vi "GetExecutionMode.vi"(8 "error in (no error)":errorcluster, 11 "absolute custom device xml file":path) -> (0 "error out":errorcluster, 2 "execution mode":T1, 3 "absolute custom device xml file":path)   [LabVIEW 2016, in "VeriStandTestUtilities.lvlib"]
uses:
  VeriStandTestUtilities.lvlib
  <vilib>/NI Veristand/Custom Device API/Custom Device Execution Mode.ctl
  <vilib>/xml/Load XML File.vi
  <vilib>/xml/Close Reference(Node).vi
  <vilib>/xml/NI_XML.lvlib
  <vilib>/NI VeriStand/Custom Device API/Custom Device API.lvlib
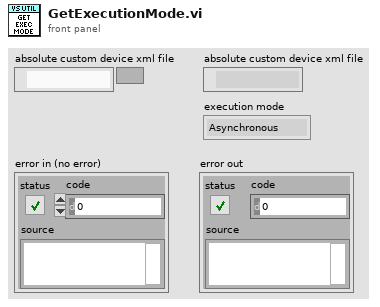
[diagram p1: front panel]
types:
  T1 = typedef "Custom Device API.lvlib/Custom Device Execution Mode.ctl" = enum16{"Asynchronous", "Inline HW Interface", "Inline Model Interface", "Inline Timing and Sync", "Asynchronous Timing and Sync"}
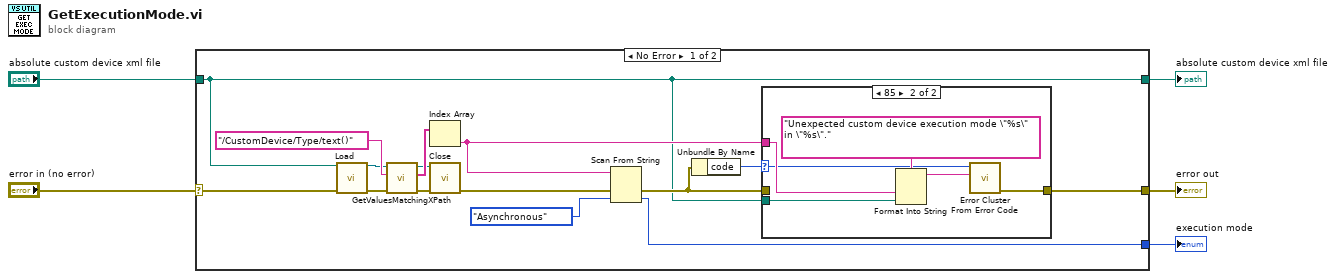
[diagram p0: block diagram]
diagram:
  n1 = case shown="No Error" "error in (no error)" {
    selector: "error in (no error)" -> [w20 w29]
    tunnel: "absolute custom device xml file" -> [w6 w28]
    tunnel: [w10 w29] -> w3
    tunnel: [w11 _] -> w2
    tunnel: [w6 w28] -> w1
    frame No Error {
      n2 = call-poly <vilib>:"Load.vi"("path to XML document"=w6, "error in (no error)"=w20) -> ("DOM document out"=w15:refnum<k20>, "error out"=w17:errorcluster)  [unwired: 11 in, 1 out]
      n3 = call "GetValuesMatchingXPath.vi"("error in (no error)"=w17, "XPath"="/CustomDevice/Type/text()", "XML refnum in"=w15) -> ("error out"=w18:errorcluster, "Values"=w16:string[], "XML refnum out"=w14:refnum<k20>)  [unwired: 6 in]
      n4 = Index Array(array=w16) -> (element=w7:string)  [unwired: 1 in]
      n5 = call-poly <vilib>:"Close.vi"("error in (no error)"=w18, "node"=w14) -> ("error out"=w12:errorcluster)  [unwired: 7 in]
      n6 = Scan From String(input string=w7, error in=w12, default 1=Custom_Device_Execution_Mode."Asynchronous" ("Execution Mode")) -> (error out=w9:errorcluster, output 1=w11:T1)  [unwired: 2 in, 2 out]
      n7 = Unbundle By Name(w9) -> ("code"=w8:i32)
      n8 = case shown="85" w8 {
        selector: w8 -> [_ w25]
        tunnel: w9 -> [w21 _]
        tunnel: [w21 w24] -> w10
        tunnel: w7 -> [_ w26]
        tunnel: w6 -> [_ w22]
        frame Default {
        }
        frame 85 {
          n9 = Format Into String(format string="Unexpected custom device execution mode \"%s\" in \"%s\"." ("error message (\"\")"), w26, w22) -> (resulting string=w23:string)  [unwired: 2 in, 1 out]
          n10 = call <vilib>:"Error Cluster From Error Code.vi"("error message (\"\")"=w23, "error code (0)"=w25) -> ("error out"=w24:errorcluster)  [unwired: 7 in]
        }
      }
    }
    frame Error {
    }
  }
  "error out" <- w3
  "execution mode" <- w2
  "absolute custom device xml file" <- w1
